vi "Get closest point on path.vi"(7 "Lookahead":dbl, 9 "index in":i32, 10 "Odometry":T1, 11 "Path in":T2[](array[typedef])) -> (2 "index out":i32, 3 "Path out":T2[](array[typedef]))   [LabVIEW 2018, in "Pure Pursuit.lvlib"]
uses:
  Pure Pursuit.lvlib
  Typedef/Path Point.ctl
  Odometry/Typedef/Odometry.ctl
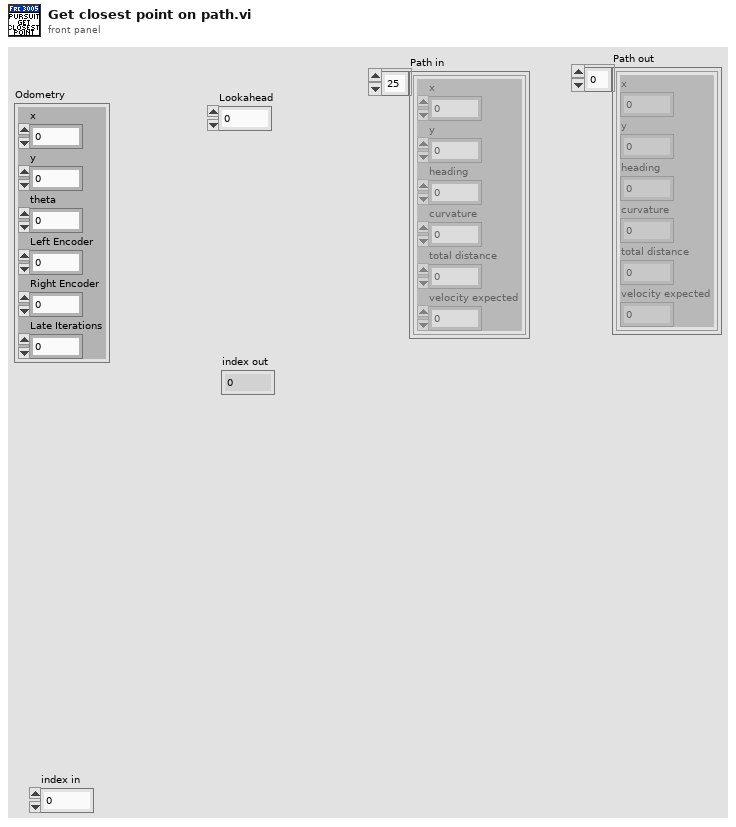
[diagram p1: front panel]
types:
  T1 = typedef "Odometry.ctl" = cluster{"x":dbl, "y":dbl, "theta":dbl, "Left Encoder":dbl, "Right Encoder":dbl, "Late Iterations":i16}
  T2 = typedef "Pure Pursuit.lvlib/Path Point.ctl" = cluster{"x":dbl, "y":dbl, "heading":dbl, "curvature":dbl, "total distance":dbl, "velocity expected":dbl}
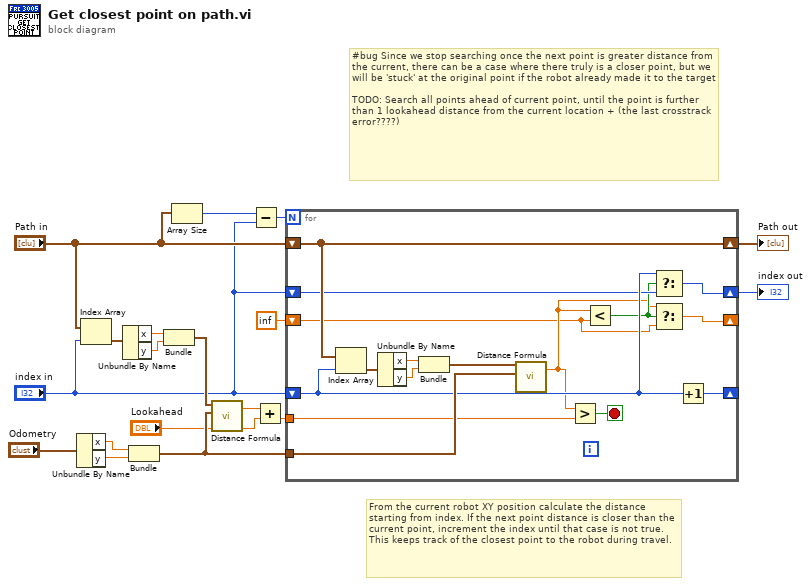
[diagram p0: block diagram]
diagram:
  # "#bug Since we stop searching once the next point is greater distance from the current, there can be a case where there truly is a closer point, but we will be 'stuck' at the original point if the robot already made it to the target\n\nTODO: Search all points ahead of current point, until the point is further than 1 lookahead distance from the current location + (the last crosstrack error????)"
  # "From the current robot XY position calculate the distance starting from index. If the next point distance is closer than the current point, increment the index until that case is not true. This keeps track of the closest point to the robot during travel."
  n1 = Unbundle By Name("Odometry") -> ("x"=w18:dbl, "y"=w17:dbl)
  n2 = Index Array(array="Path in", index="index in") -> (element=w8:T2)
  n3 = Unbundle By Name(w8) -> ("x"=w10:dbl, "y"=w9:dbl)
  n4 = Bundle("x"=w18, "y"=w17) -> (w12:cluster{"x":dbl, "y":dbl})  [unwired: 1 in]
  n5 = Bundle("x"=w10, "y"=w9) -> (w7:cluster{"x":dbl, "y":dbl})  [unwired: 1 in]
  n6 = Array Size(array="Path in") -> (size(s)=w15:i32)
  n7 = call "Distance Formula.vi"("Point2"=w12, "Point1"=w7) -> ("Distance"=w6:dbl)  [unwired: 3 in]
  n8 = Subtract(x=w15, y="index in") -> (x-y=w16:i32)
  n9 = Add(x=w6, y="Lookahead") -> (x+y=w5:dbl)
  n10 = for {
    N: w16 -> [_]
    shift-right: [w34] -> w14
    shift-left: "Path in" -> [w34]
    shift-right: [w28] -> _
    shift-left: "index in" -> [w25]
    tunnel: w12 -> [w29]
    shift-right: [w22] -> _
    shift-left: inf -> [w19]
    tunnel: w5 -> [w27]
    shift-right: [w24] -> w3
    shift-left: "index in" -> [w23]
    stop <- w26 stop-if-true
    n11 = Index Array(array=w34, index=w25) -> (element=w33:T2)
    n12 = Unbundle By Name(w33) -> ("x"=w31:dbl, "y"=w32:dbl)
    n13 = Bundle("x"=w31, "y"=w32) -> (w30:cluster{"x":dbl, "y":dbl})  [unwired: 1 in]
    n14 = call "Distance Formula.vi"("Point2"=w29, "Point1"=w30) -> ("Distance"=w20:dbl)  [unwired: 3 in]
    n15 = Greater?(x=w20, y=w27) -> (0:w26:bool)
    n16 = Less?(x=w20, y=w19) -> (x < y?=w21:bool)
    n17 = Select(t=w25, s=w21, f=w23) -> (s? t:f=w24:i32)
    n18 = Select(t=w20, s=w21, f=w19) -> (s? t:f=w22:dbl)
    n19 = Increment(x=w25) -> (x+1=w28:i32)
  }
  "index out" <- w3
  "Path out" <- w14
